vi "FTW-CodeGen-StaticLinks.vi"() -> ()   [LabVIEW 2015, in "FTW-CodeGen-StaticLinks.lvclass"]
uses:
  FTW-CodeGen-StaticLinks.lvclass
  xnode/actor/ask/FTW-CodeGen-AdaptToInputs.vi
  xnode/actor/ask/FTW-CodeGen-Bounds.vi
  xnode/actor/ask/FTW-CodeGen-Compare.vi
  xnode/actor/ask/FTW-CodeGen-DisplayName.vi
  xnode/actor/ask/FTW-CodeGen-GenerateCode.vi
  xnode/actor/ask/FTW-CodeGen-GetHelp.vi
  xnode/actor/ask/FTW-CodeGen-GetTerms.vi
  xnode/actor/ask/FTW-CodeGen-Image.vi
  xnode/actor/ask/FTW-CodeGen-Initialize.vi
  xnode/actor/ask/FTW-CodeGen-Prototype.vi
  xnode/actor/ask/FTW-CodeGen-State.ctl
  xnode/actor/ask/FTW-CodeGen-UpdateStateWithRef.vi
  xnode/actor/spawn/FTW-CodeGen-AdaptToInputs.vi
  xnode/actor/spawn/FTW-CodeGen-Bounds.vi
  xnode/actor/spawn/FTW-CodeGen-Compare.vi
  xnode/actor/spawn/FTW-CodeGen-DisplayName.vi
  xnode/actor/spawn/FTW-CodeGen-GenerateCode.vi
  xnode/actor/spawn/FTW-CodeGen-GetHelp.vi
  xnode/actor/spawn/FTW-CodeGen-GetTerms.vi
  xnode/actor/spawn/FTW-CodeGen-Image.vi
  xnode/actor/spawn/FTW-CodeGen-Initialize.vi
  xnode/actor/spawn/FTW-CodeGen-Prototype.vi
  xnode/actor/spawn/FTW-CodeGen-State.ctl
  xnode/actor/spawn/FTW-CodeGen-UpdateStateWithRef.vi
  xnode/array/shuffle/FTW-CodeGen-AdaptToInputs.vi
  xnode/array/shuffle/FTW-CodeGen-Bounds.vi
  xnode/array/shuffle/FTW-CodeGen-Compare.vi
  xnode/array/shuffle/FTW-CodeGen-DisplayName.vi
  xnode/array/shuffle/FTW-CodeGen-GenerateCode.vi
  xnode/array/shuffle/FTW-CodeGen-GetHelp.vi
  xnode/array/shuffle/FTW-CodeGen-GetTerms.vi
  xnode/array/shuffle/FTW-CodeGen-Image.vi
  xnode/array/shuffle/FTW-CodeGen-Initialize.vi
  xnode/array/shuffle/FTW-CodeGen-Prototype.vi
  xnode/array/shuffle/FTW-CodeGen-State.ctl
  xnode/array/shuffle/FTW-CodeGen-UpdateStateWithRef.vi
  xnode/dataflow/barrier/FTW-CodeGen-AdaptToInputs.vi
  xnode/dataflow/barrier/FTW-CodeGen-Bounds.vi
  xnode/dataflow/barrier/FTW-CodeGen-Compare.vi
  xnode/dataflow/barrier/FTW-CodeGen-DisplayName.vi
  xnode/dataflow/barrier/FTW-CodeGen-GenerateCode.vi
  xnode/dataflow/barrier/FTW-CodeGen-GetHelp.vi
  xnode/dataflow/barrier/FTW-CodeGen-GetTerms.vi
  xnode/dataflow/barrier/FTW-CodeGen-Image.vi
  xnode/dataflow/barrier/FTW-CodeGen-Initialize.vi
  xnode/dataflow/barrier/FTW-CodeGen-Prototype.vi
  xnode/dataflow/barrier/FTW-CodeGen-State.ctl
  xnode/dataflow/barrier/FTW-CodeGen-UpdateStateWithRef.vi
  xnode/dataflow/barrier/FTW-CodeGen-BuildMenu5.vi
  xnode/dataflow/barrier/FTW-CodeGen-GetGrowInfo.vi
  xnode/dataflow/barrier/FTW-CodeGen-OnResize2.vi
  xnode/dataflow/barrier/FTW-CodeGen-SelectMenu5.vi
  xnode/dotNET/sql/fetch/FTW-CodeGen-AdaptToInputs.vi
  xnode/dotNET/sql/fetch/FTW-CodeGen-Bounds.vi
  xnode/dotNET/sql/fetch/FTW-CodeGen-Compare.vi
  xnode/dotNET/sql/fetch/FTW-CodeGen-DisplayName.vi
  xnode/dotNET/sql/fetch/FTW-CodeGen-GenerateCode.vi
  xnode/dotNET/sql/fetch/FTW-CodeGen-GetHelp.vi
  xnode/dotNET/sql/fetch/FTW-CodeGen-GetTerms.vi
  xnode/dotNET/sql/fetch/FTW-CodeGen-Image.vi
  xnode/dotNET/sql/fetch/FTW-CodeGen-Initialize.vi
  xnode/dotNET/sql/fetch/FTW-CodeGen-Prototype.vi
  xnode/dotNET/sql/fetch/FTW-CodeGen-State.ctl
  xnode/dotNET/sql/fetch/FTW-CodeGen-UpdateStateWithRef.vi
  xnode/dotNET/sql/insert/FTW-CodeGen-AdaptToInputs.vi
  xnode/dotNET/sql/insert/FTW-CodeGen-Bounds.vi
  xnode/dotNET/sql/insert/FTW-CodeGen-Compare.vi
  xnode/dotNET/sql/insert/FTW-CodeGen-DisplayName.vi
  xnode/dotNET/sql/insert/FTW-CodeGen-GenerateCode.vi
  xnode/dotNET/sql/insert/FTW-CodeGen-GetHelp.vi
  xnode/dotNET/sql/insert/FTW-CodeGen-GetTerms.vi
  xnode/dotNET/sql/insert/FTW-CodeGen-Image.vi
  xnode/dotNET/sql/insert/FTW-CodeGen-Initialize.vi
  xnode/dotNET/sql/insert/FTW-CodeGen-Prototype.vi
  xnode/dotNET/sql/insert/FTW-CodeGen-State.ctl
  xnode/dotNET/sql/insert/FTW-CodeGen-UpdateStateWithRef.vi
  xnode/json/fetch/FTW-CodeGen-AdaptToInputs.vi
  xnode/json/fetch/FTW-CodeGen-Bounds.vi
  xnode/json/fetch/FTW-CodeGen-Compare.vi
  xnode/json/fetch/FTW-CodeGen-DisplayName.vi
  xnode/json/fetch/FTW-CodeGen-GenerateCode.vi
  xnode/json/fetch/FTW-CodeGen-GetHelp.vi
  xnode/json/fetch/FTW-CodeGen-GetTerms.vi
  xnode/json/fetch/FTW-CodeGen-Image.vi
  xnode/json/fetch/FTW-CodeGen-Initialize.vi
  xnode/json/fetch/FTW-CodeGen-Prototype.vi
  xnode/json/fetch/FTW-CodeGen-State.ctl
  xnode/json/fetch/FTW-CodeGen-UpdateStateWithRef.vi
  xnode/sqlite/fetch/FTW-CodeGen-AdaptToInputs.vi
  xnode/sqlite/fetch/FTW-CodeGen-Bounds.vi
  xnode/sqlite/fetch/FTW-CodeGen-Compare.vi
  xnode/sqlite/fetch/FTW-CodeGen-DisplayName.vi
  xnode/sqlite/fetch/FTW-CodeGen-GenerateCode.vi
  xnode/sqlite/fetch/FTW-CodeGen-GetHelp.vi
  xnode/sqlite/fetch/FTW-CodeGen-GetTerms.vi
  xnode/sqlite/fetch/FTW-CodeGen-Image.vi
  xnode/sqlite/fetch/FTW-CodeGen-Initialize.vi
  xnode/sqlite/fetch/FTW-CodeGen-Prototype.vi
  xnode/sqlite/fetch/FTW-CodeGen-State.ctl
  xnode/sqlite/fetch/FTW-CodeGen-UpdateStateWithRef.vi
  xnode/sqlite/insert/FTW-CodeGen-AdaptToInputs.vi
  xnode/sqlite/insert/FTW-CodeGen-Bounds.vi
  xnode/sqlite/insert/FTW-CodeGen-Compare.vi
  xnode/sqlite/insert/FTW-CodeGen-DisplayName.vi
  xnode/sqlite/insert/FTW-CodeGen-GenerateCode.vi
  xnode/sqlite/insert/FTW-CodeGen-GetHelp.vi
  xnode/sqlite/insert/FTW-CodeGen-GetTerms.vi
  xnode/sqlite/insert/FTW-CodeGen-Image.vi
  xnode/sqlite/insert/FTW-CodeGen-Initialize.vi
  xnode/sqlite/insert/FTW-CodeGen-Prototype.vi
  xnode/sqlite/insert/FTW-CodeGen-State.ctl
  xnode/sqlite/insert/FTW-CodeGen-UpdateStateWithRef.vi
  xnode/FTW-Actor-Ask.xnode
  xnode/FTW-Actor-Spawn.xnode
  xnode/FTW-Array-Shuffle.xnode
  xnode/FTW-Dataflow-Synchronizer.xnode
  xnode/FTW-dotNet-SQL-Fetch.xnode
  xnode/FTW-dotNet-SQL-Insert.xnode
  xnode/FTW-JSON-Fetch.xnode
  xnode/FTW-SQLite-Fetch.xnode
  xnode/FTW-SQLite-Insert.xnode
panel:
  in  "Include Dependencies?":bool=TRUE
  out "Files with static link here":path[](array[path])
  out "Files in Project but with no static link here":path[](array[path])
  # "This VI contains all static links to CodeGen and XNode source.\nIt is within a class purely because of the behavior of LVClasses to keep member VI's loaded into memory on open of the LVProject.\nKeeping this VI in memory also loads its static links into memory, enabling project operations such as \"Find All Instances\", avoiding\ndeferred compiliation in order to examine errors and linkages, and also to easily examine compile times for all VIs after clearing\nthe compiled object cache prior to running FTW-DevUtil-VIDetails.vi. Run this VI for it to examine the project to ensure it has\nstatic links to all VIs in the project."
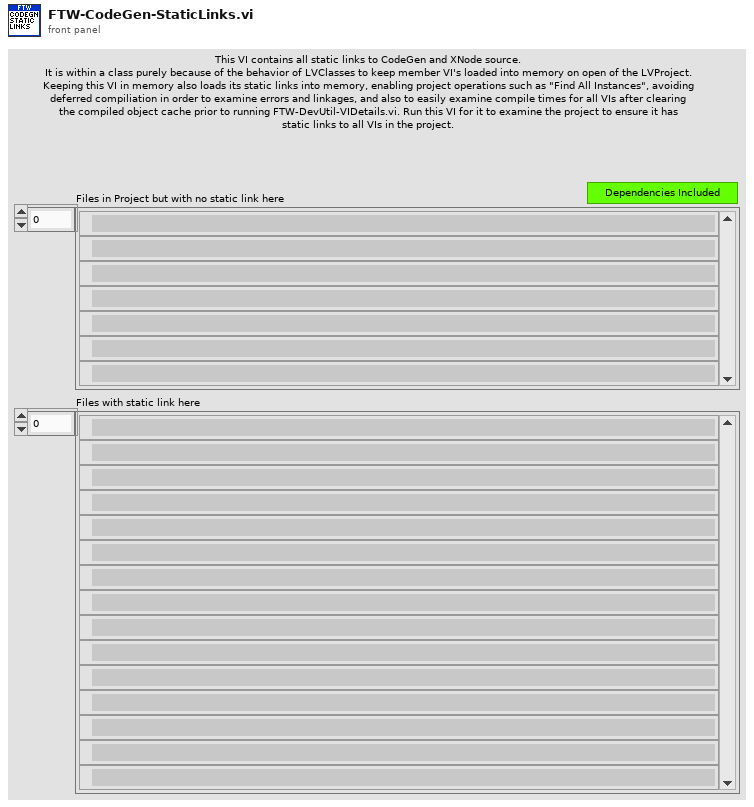
[diagram p1: front panel]
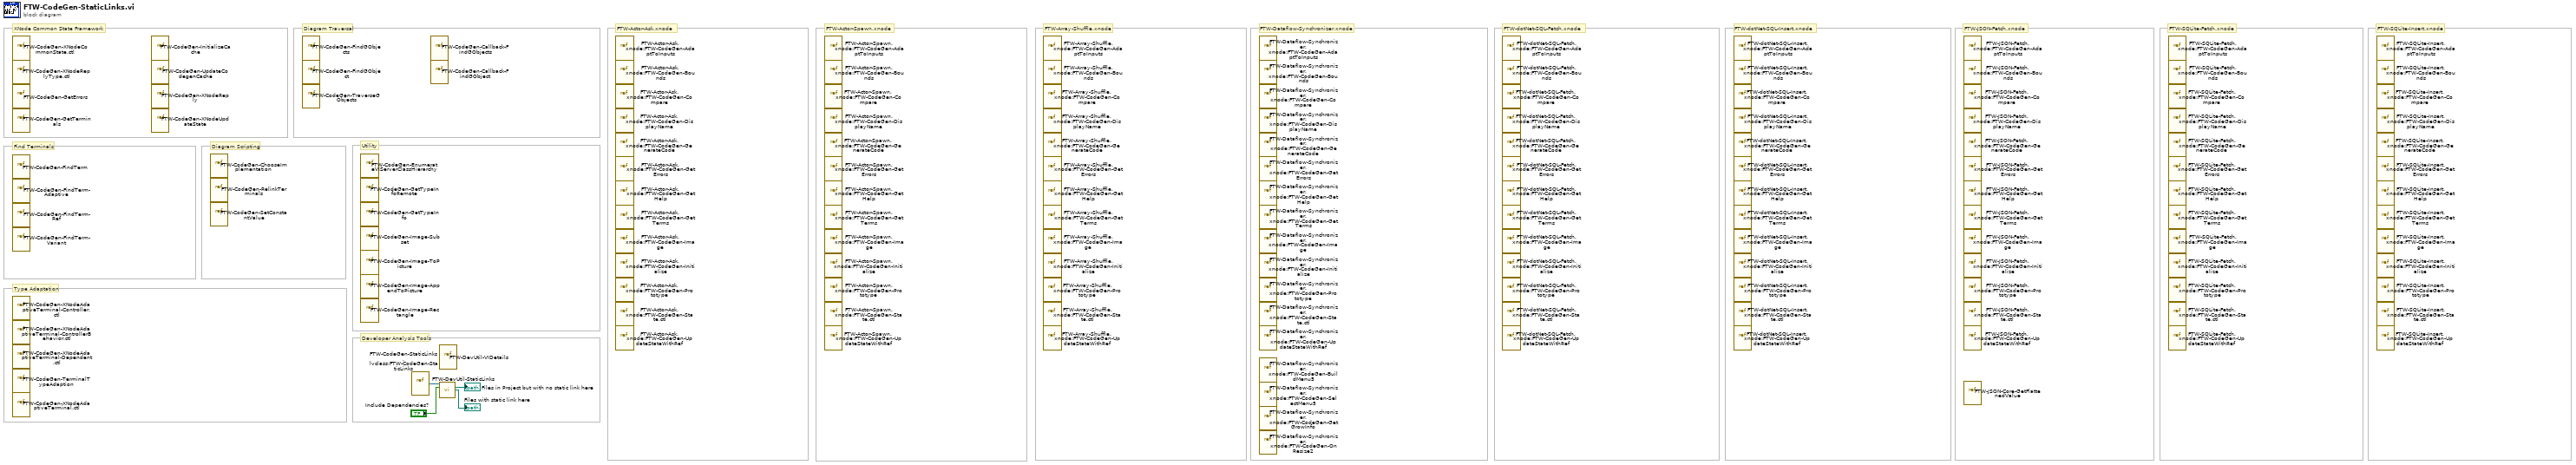
[diagram p0: block diagram]
diagram:
  # "Developer Analysis Tools"
  # "Find Terminals"
  # "FTW-SQLite-Insert.xnode"
  # "FTW-SQLite-Fetch.xnode"
  # "FTW-JSON-Fetch.xnode"
  # "FTW-dotNet-SQL-Insert.xnode"
  # "FTW-dotNet-SQL-Fetch.xnode"
  # "FTW-Dataflow-Synchronizer.xnode"
  # "FTW-Array-Shuffle.xnode"
  # "FTW-Actor-Spawn.xnode"
  # "FTW-Actor-Ask.xnode"
  # "Utility"
  # "Diagram Traversal"
  # "Diagram Scripting"
  # "XNode Common State Framework"
  # "Type Adaptation"
  n1 = vi-ref "FTW-CodeGen-XNodeCommonState.ctl"() -> ()  [unwired: 1 out]
  n2 = vi-ref "FTW-CodeGen-XNodeReplyType.ctl"() -> ()  [unwired: 1 out]
  n3 = vi-ref "FTW-CodeGen-GetErrors.vi"() -> ()  [unwired: 1 out]
  n4 = vi-ref "FTW-CodeGen-GetTerminals.vi"() -> ()  [unwired: 1 out]
  n5 = vi-ref "FTW-CodeGen-FindTerm.vi"() -> ()  [unwired: 1 out]
  n6 = vi-ref "FTW-CodeGen-FindTerm-Adaptive.vi"() -> ()  [unwired: 1 out]
  n7 = vi-ref "FTW-CodeGen-FindTerm-Ref.vi"() -> ()  [unwired: 1 out]
  n8 = vi-ref "FTW-CodeGen-FindTerm-Variant.vi"() -> ()  [unwired: 1 out]
  n9 = vi-ref "FTW-CodeGen-XNodeAdaptiveTerminal-Controller.ctl"() -> ()  [unwired: 1 out]
  n10 = vi-ref "FTW-CodeGen-XNodeAdaptiveTerminal-ControllerBehavior.ctl"() -> ()  [unwired: 1 out]
  n11 = vi-ref "FTW-CodeGen-XNodeAdaptiveTerminal-Dependent.ctl"() -> ()  [unwired: 1 out]
  n12 = vi-ref "FTW-CodeGen-TerminalTypeAdaption.vi"() -> ()  [unwired: 1 out]
  n13 = vi-ref "FTW-CodeGen-XNodeAdaptiveTerminal.ctl"() -> ()  [unwired: 1 out]
  n14 = vi-ref "FTW-CodeGen-InitializeCache.vi"() -> ()  [unwired: 1 out]
  n15 = vi-ref "FTW-CodeGen-UpdateCodegenCache.vi"() -> ()  [unwired: 1 out]
  n16 = vi-ref "FTW-CodeGen-XNodeReply.vi"() -> ()  [unwired: 1 out]
  n17 = vi-ref "FTW-CodeGen-XNodeUpdateState.vi"() -> ()  [unwired: 1 out]
  n18 = vi-ref "FTW-CodeGen-ChooseImplementation.vi"() -> ()  [unwired: 1 out]
  n19 = vi-ref "FTW-CodeGen-RelinkTerminals.vi"() -> ()  [unwired: 1 out]
  n20 = vi-ref "FTW-CodeGen-SetConstantValue.vi"() -> ()  [unwired: 1 out]
  n21 = vi-ref "FTW-CodeGen-FindGObjects.vi"() -> ()  [unwired: 1 out]
  n22 = vi-ref "FTW-CodeGen-FindGObject.vi"() -> ()  [unwired: 1 out]
  n23 = vi-ref "FTW-CodeGen-TraverseGObjects.vi"() -> ()  [unwired: 1 out]
  n24 = vi-ref "FTW-CodeGen-EnumerateVIServerClassHierarchy.vi"() -> ()  [unwired: 1 out]
  n25 = vi-ref "FTW-CodeGen-GetTypeInfoRemote.vi"() -> ()  [unwired: 1 out]
  n26 = vi-ref "FTW-CodeGen-GetTypeInfo.vi"() -> ()  [unwired: 1 out]
  n27 = vi-ref "FTW-CodeGen-Image-Subset.vi"() -> ()  [unwired: 1 out]
  n28 = vi-ref "FTW-CodeGen-Image-ToPicture.vi"() -> ()  [unwired: 1 out]
  n29 = vi-ref "FTW-CodeGen-Image-AppendToPicture.vi"() -> ()  [unwired: 1 out]
  n30 = vi-ref "FTW-CodeGen-Image-Rectangle.vi"() -> ()  [unwired: 1 out]
  n31 = vi-ref "FTW-CodeGen-StaticLinks.lvclass:FTW-CodeGen-StaticLinks.vi"() -> (w4:refnum<vi>)
  n32 = vi-ref "FTW-CodeGen-Callback-FindGObjects.vi"() -> ()  [unwired: 1 out]
  n33 = vi-ref "FTW-CodeGen-Callback-FindGObject.vi"() -> ()  [unwired: 1 out]
  n34 = vi-ref "FTW-DevUtil-VIDetails.vi"() -> ()  [unwired: 1 out]
  n35 = call "FTW-DevUtil-StaticLinks.vi"("VI Ref"=w4, "Include Dependencies?"="Include Dependencies?") -> ("Files in Project but with no static link here"=→"Files in Project but with no static link here":path[], "Files with static link here"=→"Files with static link here":path[])  [unwired: 11 in, 1 out]
  n36 = vi-ref "FTW-Actor-Ask.xnode:FTW-CodeGen-AdaptToInputs.vi"() -> ()  [unwired: 1 out]
  n37 = vi-ref "FTW-Actor-Ask.xnode:FTW-CodeGen-Bounds.vi"() -> ()  [unwired: 1 out]
  n38 = vi-ref "FTW-Actor-Ask.xnode:FTW-CodeGen-Compare.vi"() -> ()  [unwired: 1 out]
  n39 = vi-ref "FTW-Actor-Ask.xnode:FTW-CodeGen-DisplayName.vi"() -> ()  [unwired: 1 out]
  n40 = vi-ref "FTW-Actor-Ask.xnode:FTW-CodeGen-GenerateCode.vi"() -> ()  [unwired: 1 out]
  n41 = vi-ref "FTW-Actor-Ask.xnode:FTW-CodeGen-GetErrors.vi"() -> ()  [unwired: 1 out]
  n42 = vi-ref "FTW-Actor-Ask.xnode:FTW-CodeGen-GetHelp.vi"() -> ()  [unwired: 1 out]
  n43 = vi-ref "FTW-Actor-Ask.xnode:FTW-CodeGen-GetTerms.vi"() -> ()  [unwired: 1 out]
  n44 = vi-ref "FTW-Actor-Ask.xnode:FTW-CodeGen-Image.vi"() -> ()  [unwired: 1 out]
  n45 = vi-ref "FTW-Actor-Ask.xnode:FTW-CodeGen-Initialize.vi"() -> ()  [unwired: 1 out]
  n46 = vi-ref "FTW-Actor-Ask.xnode:FTW-CodeGen-Prototype.vi"() -> ()  [unwired: 1 out]
  n47 = vi-ref "FTW-Actor-Ask.xnode:FTW-CodeGen-State.ctl"() -> ()  [unwired: 1 out]
  n48 = vi-ref "FTW-Actor-Ask.xnode:FTW-CodeGen-UpdateStateWithRef.vi"() -> ()  [unwired: 1 out]
  n49 = vi-ref "FTW-Actor-Spawn.xnode:FTW-CodeGen-AdaptToInputs.vi"() -> ()  [unwired: 1 out]
  n50 = vi-ref "FTW-Actor-Spawn.xnode:FTW-CodeGen-Bounds.vi"() -> ()  [unwired: 1 out]
  n51 = vi-ref "FTW-Actor-Spawn.xnode:FTW-CodeGen-Compare.vi"() -> ()  [unwired: 1 out]
  n52 = vi-ref "FTW-Actor-Spawn.xnode:FTW-CodeGen-DisplayName.vi"() -> ()  [unwired: 1 out]
  n53 = vi-ref "FTW-Actor-Spawn.xnode:FTW-CodeGen-GenerateCode.vi"() -> ()  [unwired: 1 out]
  n54 = vi-ref "FTW-Actor-Spawn.xnode:FTW-CodeGen-GetErrors.vi"() -> ()  [unwired: 1 out]
  n55 = vi-ref "FTW-Actor-Spawn.xnode:FTW-CodeGen-GetHelp.vi"() -> ()  [unwired: 1 out]
  n56 = vi-ref "FTW-Actor-Spawn.xnode:FTW-CodeGen-GetTerms.vi"() -> ()  [unwired: 1 out]
  n57 = vi-ref "FTW-Actor-Spawn.xnode:FTW-CodeGen-Image.vi"() -> ()  [unwired: 1 out]
  n58 = vi-ref "FTW-Actor-Spawn.xnode:FTW-CodeGen-Initialize.vi"() -> ()  [unwired: 1 out]
  n59 = vi-ref "FTW-Actor-Spawn.xnode:FTW-CodeGen-Prototype.vi"() -> ()  [unwired: 1 out]
  n60 = vi-ref "FTW-Actor-Spawn.xnode:FTW-CodeGen-State.ctl"() -> ()  [unwired: 1 out]
  n61 = vi-ref "FTW-Actor-Spawn.xnode:FTW-CodeGen-UpdateStateWithRef.vi"() -> ()  [unwired: 1 out]
  n62 = vi-ref "FTW-Array-Shuffle.xnode:FTW-CodeGen-AdaptToInputs.vi"() -> ()  [unwired: 1 out]
  n63 = vi-ref "FTW-Array-Shuffle.xnode:FTW-CodeGen-Bounds.vi"() -> ()  [unwired: 1 out]
  n64 = vi-ref "FTW-Array-Shuffle.xnode:FTW-CodeGen-Compare.vi"() -> ()  [unwired: 1 out]
  n65 = vi-ref "FTW-Array-Shuffle.xnode:FTW-CodeGen-DisplayName.vi"() -> ()  [unwired: 1 out]
  n66 = vi-ref "FTW-Array-Shuffle.xnode:FTW-CodeGen-GenerateCode.vi"() -> ()  [unwired: 1 out]
  n67 = vi-ref "FTW-Array-Shuffle.xnode:FTW-CodeGen-GetErrors.vi"() -> ()  [unwired: 1 out]
  n68 = vi-ref "FTW-Array-Shuffle.xnode:FTW-CodeGen-GetHelp.vi"() -> ()  [unwired: 1 out]
  n69 = vi-ref "FTW-Array-Shuffle.xnode:FTW-CodeGen-GetTerms.vi"() -> ()  [unwired: 1 out]
  n70 = vi-ref "FTW-Array-Shuffle.xnode:FTW-CodeGen-Image.vi"() -> ()  [unwired: 1 out]
  n71 = vi-ref "FTW-Array-Shuffle.xnode:FTW-CodeGen-Initialize.vi"() -> ()  [unwired: 1 out]
  n72 = vi-ref "FTW-Array-Shuffle.xnode:FTW-CodeGen-Prototype.vi"() -> ()  [unwired: 1 out]
  n73 = vi-ref "FTW-Array-Shuffle.xnode:FTW-CodeGen-State.ctl"() -> ()  [unwired: 1 out]
  n74 = vi-ref "FTW-Array-Shuffle.xnode:FTW-CodeGen-UpdateStateWithRef.vi"() -> ()  [unwired: 1 out]
  n75 = vi-ref "FTW-Dataflow-Synchronizer.xnode:FTW-CodeGen-AdaptToInputs.vi"() -> ()  [unwired: 1 out]
  n76 = vi-ref "FTW-Dataflow-Synchronizer.xnode:FTW-CodeGen-Bounds.vi"() -> ()  [unwired: 1 out]
  n77 = vi-ref "FTW-Dataflow-Synchronizer.xnode:FTW-CodeGen-Compare.vi"() -> ()  [unwired: 1 out]
  n78 = vi-ref "FTW-Dataflow-Synchronizer.xnode:FTW-CodeGen-DisplayName.vi"() -> ()  [unwired: 1 out]
  n79 = vi-ref "FTW-Dataflow-Synchronizer.xnode:FTW-CodeGen-GenerateCode.vi"() -> ()  [unwired: 1 out]
  n80 = vi-ref "FTW-Dataflow-Synchronizer.xnode:FTW-CodeGen-GetErrors.vi"() -> ()  [unwired: 1 out]
  n81 = vi-ref "FTW-Dataflow-Synchronizer.xnode:FTW-CodeGen-GetHelp.vi"() -> ()  [unwired: 1 out]
  n82 = vi-ref "FTW-Dataflow-Synchronizer.xnode:FTW-CodeGen-GetTerms.vi"() -> ()  [unwired: 1 out]
  n83 = vi-ref "FTW-Dataflow-Synchronizer.xnode:FTW-CodeGen-Image.vi"() -> ()  [unwired: 1 out]
  n84 = vi-ref "FTW-Dataflow-Synchronizer.xnode:FTW-CodeGen-Initialize.vi"() -> ()  [unwired: 1 out]
  n85 = vi-ref "FTW-Dataflow-Synchronizer.xnode:FTW-CodeGen-Prototype.vi"() -> ()  [unwired: 1 out]
  n86 = vi-ref "FTW-Dataflow-Synchronizer.xnode:FTW-CodeGen-State.ctl"() -> ()  [unwired: 1 out]
  n87 = vi-ref "FTW-Dataflow-Synchronizer.xnode:FTW-CodeGen-UpdateStateWithRef.vi"() -> ()  [unwired: 1 out]
  n88 = vi-ref "FTW-Dataflow-Synchronizer.xnode:FTW-CodeGen-BuildMenu5.vi"() -> ()  [unwired: 1 out]
  n89 = vi-ref "FTW-Dataflow-Synchronizer.xnode:FTW-CodeGen-SelectMenu5.vi"() -> ()  [unwired: 1 out]
  n90 = vi-ref "FTW-Dataflow-Synchronizer.xnode:FTW-CodeGen-GetGrowInfo.vi"() -> ()  [unwired: 1 out]
  n91 = vi-ref "FTW-Dataflow-Synchronizer.xnode:FTW-CodeGen-OnResize2.vi"() -> ()  [unwired: 1 out]
  n92 = vi-ref "FTW-dotNet-SQL-Fetch.xnode:FTW-CodeGen-AdaptToInputs.vi"() -> ()  [unwired: 1 out]
  n93 = vi-ref "FTW-dotNet-SQL-Fetch.xnode:FTW-CodeGen-Bounds.vi"() -> ()  [unwired: 1 out]
  n94 = vi-ref "FTW-dotNet-SQL-Fetch.xnode:FTW-CodeGen-Compare.vi"() -> ()  [unwired: 1 out]
  n95 = vi-ref "FTW-dotNet-SQL-Fetch.xnode:FTW-CodeGen-DisplayName.vi"() -> ()  [unwired: 1 out]
  n96 = vi-ref "FTW-dotNet-SQL-Fetch.xnode:FTW-CodeGen-GenerateCode.vi"() -> ()  [unwired: 1 out]
  n97 = vi-ref "FTW-dotNet-SQL-Fetch.xnode:FTW-CodeGen-GetErrors.vi"() -> ()  [unwired: 1 out]
  n98 = vi-ref "FTW-dotNet-SQL-Fetch.xnode:FTW-CodeGen-GetHelp.vi"() -> ()  [unwired: 1 out]
  n99 = vi-ref "FTW-dotNet-SQL-Fetch.xnode:FTW-CodeGen-GetTerms.vi"() -> ()  [unwired: 1 out]
  n100 = vi-ref "FTW-dotNet-SQL-Fetch.xnode:FTW-CodeGen-Image.vi"() -> ()  [unwired: 1 out]
  n101 = vi-ref "FTW-dotNet-SQL-Fetch.xnode:FTW-CodeGen-Initialize.vi"() -> ()  [unwired: 1 out]
  n102 = vi-ref "FTW-dotNet-SQL-Fetch.xnode:FTW-CodeGen-Prototype.vi"() -> ()  [unwired: 1 out]
  n103 = vi-ref "FTW-dotNet-SQL-Fetch.xnode:FTW-CodeGen-State.ctl"() -> ()  [unwired: 1 out]
  n104 = vi-ref "FTW-dotNet-SQL-Fetch.xnode:FTW-CodeGen-UpdateStateWithRef.vi"() -> ()  [unwired: 1 out]
  n105 = vi-ref "FTW-dotNet-SQL-Insert.xnode:FTW-CodeGen-AdaptToInputs.vi"() -> ()  [unwired: 1 out]
  n106 = vi-ref "FTW-dotNet-SQL-Insert.xnode:FTW-CodeGen-Bounds.vi"() -> ()  [unwired: 1 out]
  n107 = vi-ref "FTW-dotNet-SQL-Insert.xnode:FTW-CodeGen-Compare.vi"() -> ()  [unwired: 1 out]
  n108 = vi-ref "FTW-dotNet-SQL-Insert.xnode:FTW-CodeGen-DisplayName.vi"() -> ()  [unwired: 1 out]
  n109 = vi-ref "FTW-dotNet-SQL-Insert.xnode:FTW-CodeGen-GenerateCode.vi"() -> ()  [unwired: 1 out]
  n110 = vi-ref "FTW-dotNet-SQL-Insert.xnode:FTW-CodeGen-GetErrors.vi"() -> ()  [unwired: 1 out]
  n111 = vi-ref "FTW-dotNet-SQL-Insert.xnode:FTW-CodeGen-GetHelp.vi"() -> ()  [unwired: 1 out]
  n112 = vi-ref "FTW-dotNet-SQL-Insert.xnode:FTW-CodeGen-GetTerms.vi"() -> ()  [unwired: 1 out]
  n113 = vi-ref "FTW-dotNet-SQL-Insert.xnode:FTW-CodeGen-Image.vi"() -> ()  [unwired: 1 out]
  n114 = vi-ref "FTW-dotNet-SQL-Insert.xnode:FTW-CodeGen-Initialize.vi"() -> ()  [unwired: 1 out]
  n115 = vi-ref "FTW-dotNet-SQL-Insert.xnode:FTW-CodeGen-Prototype.vi"() -> ()  [unwired: 1 out]
  n116 = vi-ref "FTW-dotNet-SQL-Insert.xnode:FTW-CodeGen-State.ctl"() -> ()  [unwired: 1 out]
  n117 = vi-ref "FTW-dotNet-SQL-Insert.xnode:FTW-CodeGen-UpdateStateWithRef.vi"() -> ()  [unwired: 1 out]
  n118 = vi-ref "FTW-JSON-Fetch.xnode:FTW-CodeGen-AdaptToInputs.vi"() -> ()  [unwired: 1 out]
  n119 = vi-ref "FTW-JSON-Fetch.xnode:FTW-CodeGen-Bounds.vi"() -> ()  [unwired: 1 out]
  n120 = vi-ref "FTW-JSON-Fetch.xnode:FTW-CodeGen-Compare.vi"() -> ()  [unwired: 1 out]
  n121 = vi-ref "FTW-JSON-Fetch.xnode:FTW-CodeGen-DisplayName.vi"() -> ()  [unwired: 1 out]
  n122 = vi-ref "FTW-JSON-Fetch.xnode:FTW-CodeGen-GenerateCode.vi"() -> ()  [unwired: 1 out]
  n123 = vi-ref "FTW-JSON-Fetch.xnode:FTW-CodeGen-GetErrors.vi"() -> ()  [unwired: 1 out]
  n124 = vi-ref "FTW-JSON-Fetch.xnode:FTW-CodeGen-GetHelp.vi"() -> ()  [unwired: 1 out]
  n125 = vi-ref "FTW-JSON-Fetch.xnode:FTW-CodeGen-GetTerms.vi"() -> ()  [unwired: 1 out]
  n126 = vi-ref "FTW-JSON-Fetch.xnode:FTW-CodeGen-Image.vi"() -> ()  [unwired: 1 out]
  n127 = vi-ref "FTW-JSON-Fetch.xnode:FTW-CodeGen-Initialize.vi"() -> ()  [unwired: 1 out]
  n128 = vi-ref "FTW-JSON-Fetch.xnode:FTW-CodeGen-Prototype.vi"() -> ()  [unwired: 1 out]
  n129 = vi-ref "FTW-JSON-Fetch.xnode:FTW-CodeGen-State.ctl"() -> ()  [unwired: 1 out]
  n130 = vi-ref "FTW-JSON-Fetch.xnode:FTW-CodeGen-UpdateStateWithRef.vi"() -> ()  [unwired: 1 out]
  n131 = vi-ref "FTW-JSON-Core-GetFlattenedValue.vi"() -> ()  [unwired: 1 out]
  n132 = vi-ref "FTW-SQLite-Fetch.xnode:FTW-CodeGen-AdaptToInputs.vi"() -> ()  [unwired: 1 out]
  n133 = vi-ref "FTW-SQLite-Fetch.xnode:FTW-CodeGen-Bounds.vi"() -> ()  [unwired: 1 out]
  n134 = vi-ref "FTW-SQLite-Fetch.xnode:FTW-CodeGen-Compare.vi"() -> ()  [unwired: 1 out]
  n135 = vi-ref "FTW-SQLite-Fetch.xnode:FTW-CodeGen-DisplayName.vi"() -> ()  [unwired: 1 out]
  n136 = vi-ref "FTW-SQLite-Fetch.xnode:FTW-CodeGen-GenerateCode.vi"() -> ()  [unwired: 1 out]
  n137 = vi-ref "FTW-SQLite-Fetch.xnode:FTW-CodeGen-GetErrors.vi"() -> ()  [unwired: 1 out]
  n138 = vi-ref "FTW-SQLite-Fetch.xnode:FTW-CodeGen-GetHelp.vi"() -> ()  [unwired: 1 out]
  n139 = vi-ref "FTW-SQLite-Fetch.xnode:FTW-CodeGen-GetTerms.vi"() -> ()  [unwired: 1 out]
  n140 = vi-ref "FTW-SQLite-Fetch.xnode:FTW-CodeGen-Image.vi"() -> ()  [unwired: 1 out]
  n141 = vi-ref "FTW-SQLite-Fetch.xnode:FTW-CodeGen-Initialize.vi"() -> ()  [unwired: 1 out]
  n142 = vi-ref "FTW-SQLite-Fetch.xnode:FTW-CodeGen-Prototype.vi"() -> ()  [unwired: 1 out]
  n143 = vi-ref "FTW-SQLite-Fetch.xnode:FTW-CodeGen-State.ctl"() -> ()  [unwired: 1 out]
  n144 = vi-ref "FTW-SQLite-Fetch.xnode:FTW-CodeGen-UpdateStateWithRef.vi"() -> ()  [unwired: 1 out]
  n145 = vi-ref "FTW-SQLite-Insert.xnode:FTW-CodeGen-AdaptToInputs.vi"() -> ()  [unwired: 1 out]
  n146 = vi-ref "FTW-SQLite-Insert.xnode:FTW-CodeGen-Bounds.vi"() -> ()  [unwired: 1 out]
  n147 = vi-ref "FTW-SQLite-Insert.xnode:FTW-CodeGen-Compare.vi"() -> ()  [unwired: 1 out]
  n148 = vi-ref "FTW-SQLite-Insert.xnode:FTW-CodeGen-DisplayName.vi"() -> ()  [unwired: 1 out]
  n149 = vi-ref "FTW-SQLite-Insert.xnode:FTW-CodeGen-GenerateCode.vi"() -> ()  [unwired: 1 out]
  n150 = vi-ref "FTW-SQLite-Insert.xnode:FTW-CodeGen-GetErrors.vi"() -> ()  [unwired: 1 out]
  n151 = vi-ref "FTW-SQLite-Insert.xnode:FTW-CodeGen-GetHelp.vi"() -> ()  [unwired: 1 out]
  n152 = vi-ref "FTW-SQLite-Insert.xnode:FTW-CodeGen-GetTerms.vi"() -> ()  [unwired: 1 out]
  n153 = vi-ref "FTW-SQLite-Insert.xnode:FTW-CodeGen-Image.vi"() -> ()  [unwired: 1 out]
  n154 = vi-ref "FTW-SQLite-Insert.xnode:FTW-CodeGen-Initialize.vi"() -> ()  [unwired: 1 out]
  n155 = vi-ref "FTW-SQLite-Insert.xnode:FTW-CodeGen-Prototype.vi"() -> ()  [unwired: 1 out]
  n156 = vi-ref "FTW-SQLite-Insert.xnode:FTW-CodeGen-State.ctl"() -> ()  [unwired: 1 out]
  n157 = vi-ref "FTW-SQLite-Insert.xnode:FTW-CodeGen-UpdateStateWithRef.vi"() -> ()  [unwired: 1 out]
